vi "SRV_JPEG Filepath_Camera.vi"(2 "Dir path for JPEG file":path) -> (7 "JPEG Filepath":path)   [LabVIEW 2014]
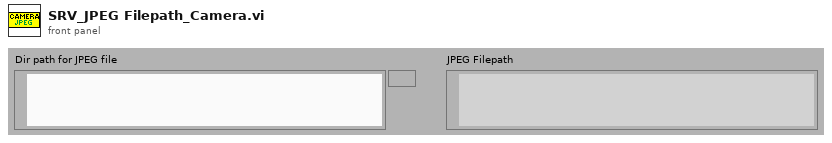
[diagram p1: front panel]
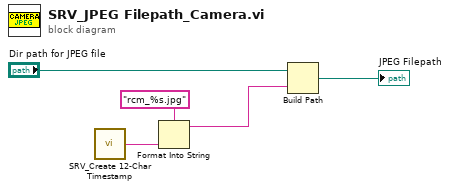
[diagram p0: block diagram]
diagram:
  n1 = call "SRV_Create 12-Char Timestamp.vi"() -> ("Timestamp String"=w2:string)  [unwired: 15 in]
  n2 = Format Into String(format string="rcm_%s.jpg", w2) -> (resulting string=w1:string)  [unwired: 2 in, 1 out]
  n3 = Build Path(base path="Dir path for JPEG file", name or relative path=w1) -> (appended path=→"JPEG Filepath":path)
